vi "communication manager.vi"() -> ()   [LabVIEW 2018]
uses:
  socket SUB/socket SUB.lvclass
  C:/Users/devstaff/sparc4/s4gui/Versao ZeroMQ REQ-REP/SPARC4_GUI -v1.0.8 - com pacote communication manager/communication-manager/Socket/Socket.lvclass
  socket PUB/socket PUB.lvclass
  socket REQ/socket REQ.lvclass
  RxTx/CM_RxTx.lvclass
  <vilib>/addons/zeromq/zmq_context.lvclass
  Socket/Socket.lvclass
panel:
  in  "socket REQ":refnum<class "socket REQ.lvclass">
  out "error out":errorcluster
  in  "socket PUB.lvclass":refnum<class "socket PUB.lvclass">
  in  "socket SUB.lvclass":refnum<class "socket SUB.lvclass">
  # "Communication Manager of S4CCS"
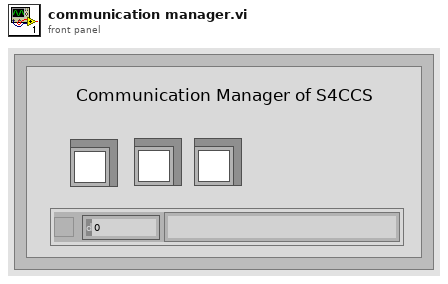
[diagram p1: front panel]
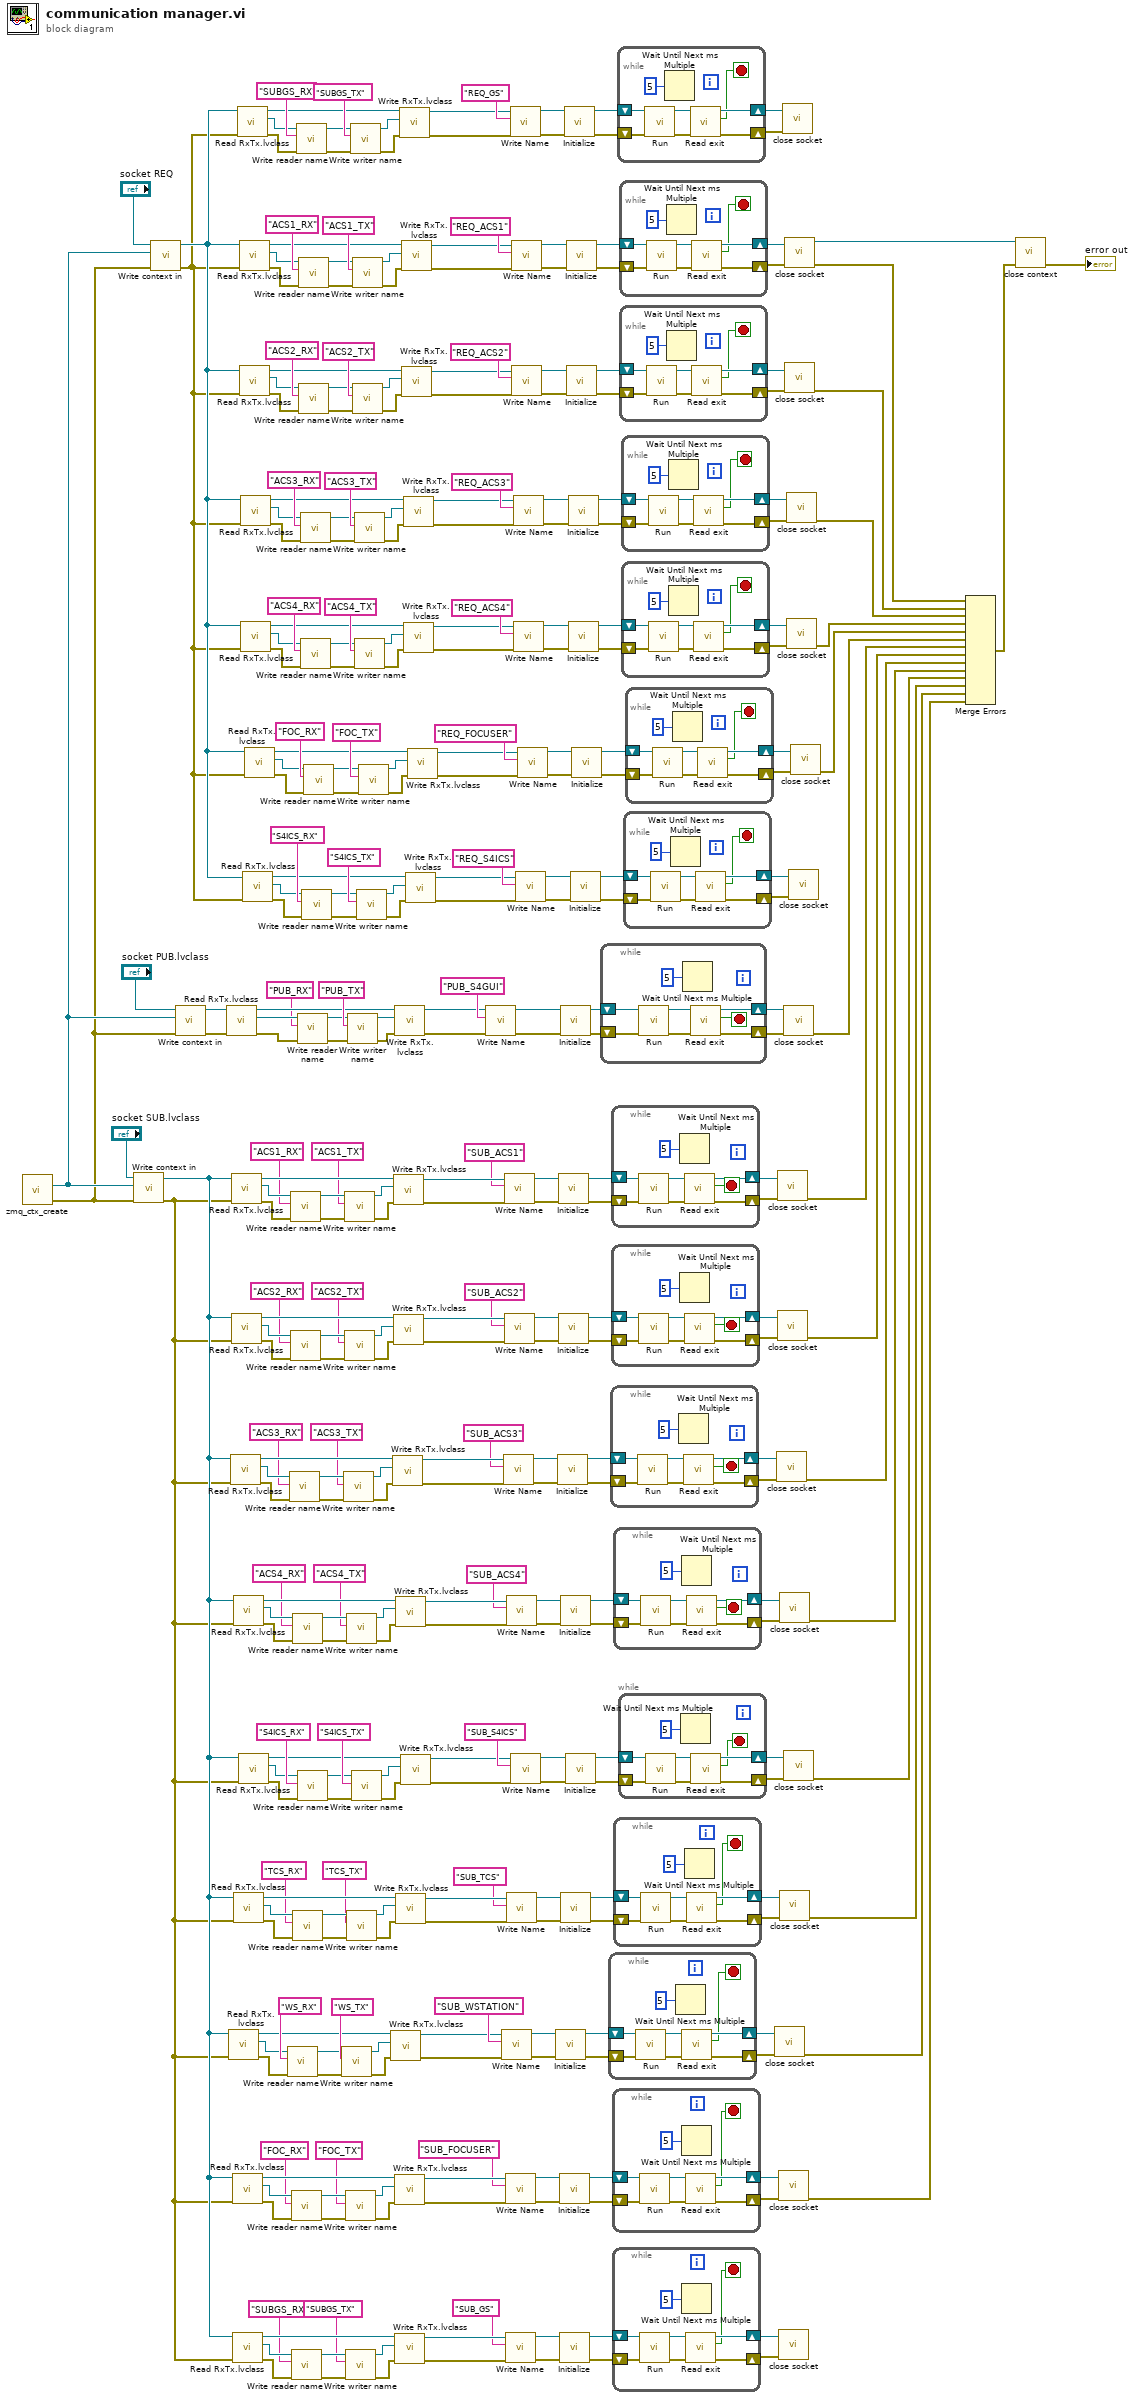
[diagram p0: block diagram]
diagram:
  n1 = call <vilib>:"zmq_ctx_create.vi"() -> ("error out"=w41:errorcluster, "context out"=w42:refnum<class "zmq_context.lvclass">)  [unwired: 4 in]
  n2 = call-dynamic "Write context in.vi"("error in (no error)"=w41, "zeromq.lvlib:ZeroMQ Context"=w42, "Socket in"="socket SUB.lvclass") -> ("error out"=w21:errorcluster, "Socket out"=w22:refnum<class "socket SUB.lvclass">)  [unwired: 7 in]
  n3 = call-dynamic "Write context in.vi"("error in (no error)"=w41, "zeromq.lvlib:ZeroMQ Context"=w42, "Socket in"="socket REQ") -> ("error out"=w1:errorcluster, "Socket out"=w2:refnum<class "socket REQ.lvclass">)  [unwired: 7 in]
  n4 = call-dynamic "Write context in.vi"("error in (no error)"=w41, "zeromq.lvlib:ZeroMQ Context"=w42, "Socket in"="socket PUB.lvclass") -> ("error out"=w199:errorcluster, "Socket out"=w200:refnum<class "socket PUB.lvclass">)  [unwired: 7 in]
  n5 = call-dynamic "Read RxTx.lvclass.vi"("error in (no error)"=w199, "Socket in"=w200) -> ("error out"=w305:errorcluster, "RxTx.lvclass"=w309:refnum<class "CM_RxTx.lvclass">, "Socket out"=w306:refnum<class "socket PUB.lvclass">)  [unwired: 7 in]
  n6 = call-dynamic "Read RxTx.lvclass.vi"("error in (no error)"=w21, "Socket in"=w22) -> ("error out"=w240:errorcluster, "RxTx.lvclass"=w244:refnum<class "CM_RxTx.lvclass">, "Socket out"=w241:refnum<class "socket SUB.lvclass">)  [unwired: 7 in]
  n7 = call-dynamic "Read RxTx.lvclass.vi"("error in (no error)"=w21, "Socket in"=w22) -> ("error out"=w109:errorcluster, "RxTx.lvclass"=w105:refnum<class "CM_RxTx.lvclass">, "Socket out"=w108:refnum<class "socket SUB.lvclass">)  [unwired: 7 in]
  n8 = call-dynamic "Read RxTx.lvclass.vi"("error in (no error)"=w21, "Socket in"=w22) -> ("error out"=w287:errorcluster, "RxTx.lvclass"=w283:refnum<class "CM_RxTx.lvclass">, "Socket out"=w286:refnum<class "socket SUB.lvclass">)  [unwired: 7 in]
  n9 = call-dynamic "Read RxTx.lvclass.vi"("error in (no error)"=w21, "Socket in"=w22) -> ("error out"=w127:errorcluster, "RxTx.lvclass"=w123:refnum<class "CM_RxTx.lvclass">, "Socket out"=w126:refnum<class "socket SUB.lvclass">)  [unwired: 7 in]
  n10 = call-dynamic "Read RxTx.lvclass.vi"("error in (no error)"=w21, "Socket in"=w22) -> ("error out"=w221:errorcluster, "RxTx.lvclass"=w217:refnum<class "CM_RxTx.lvclass">, "Socket out"=w220:refnum<class "socket SUB.lvclass">)  [unwired: 7 in]
  n11 = call-dynamic "Read RxTx.lvclass.vi"("error in (no error)"=w21, "Socket in"=w22) -> ("error out"=w31:errorcluster, "RxTx.lvclass"=w27:refnum<class "CM_RxTx.lvclass">, "Socket out"=w30:refnum<class "socket SUB.lvclass">)  [unwired: 7 in]
  n12 = call-dynamic "Read RxTx.lvclass.vi"("error in (no error)"=w21, "Socket in"=w22) -> ("error out"=w91:errorcluster, "RxTx.lvclass"=w87:refnum<class "CM_RxTx.lvclass">, "Socket out"=w90:refnum<class "socket SUB.lvclass">)  [unwired: 7 in]
  n13 = call-dynamic "Read RxTx.lvclass.vi"("error in (no error)"=w21, "Socket in"=w22) -> ("error out"=w253:errorcluster, "RxTx.lvclass"=w249:refnum<class "CM_RxTx.lvclass">, "Socket out"=w252:refnum<class "socket SUB.lvclass">)  [unwired: 7 in]
  n14 = call-dynamic "Read RxTx.lvclass.vi"("error in (no error)"=w1, "Socket in"=w2) -> ("error out"=w14:errorcluster, "RxTx.lvclass"=w18:refnum<class "CM_RxTx.lvclass">, "Socket out"=w15:refnum<class "socket REQ.lvclass">)  [unwired: 7 in]
  n15 = call-dynamic "Read RxTx.lvclass.vi"("error in (no error)"=w21, "Socket in"=w22) -> ("error out"=w272:errorcluster, "RxTx.lvclass"=w276:refnum<class "CM_RxTx.lvclass">, "Socket out"=w273:refnum<class "socket SUB.lvclass">)  [unwired: 7 in]
  n16 = call-dynamic "Read RxTx.lvclass.vi"("error in (no error)"=w1, "Socket in"=w2) -> ("error out"=w327:errorcluster, "RxTx.lvclass"=w331:refnum<class "CM_RxTx.lvclass">, "Socket out"=w328:refnum<class "socket REQ.lvclass">)  [unwired: 7 in]
  n17 = call-dynamic "Read RxTx.lvclass.vi"("error in (no error)"=w1, "Socket in"=w2) -> ("error out"=w188:errorcluster, "RxTx.lvclass"=w192:refnum<class "CM_RxTx.lvclass">, "Socket out"=w189:refnum<class "socket REQ.lvclass">)  [unwired: 7 in]
  n18 = call-dynamic "Read RxTx.lvclass.vi"("error in (no error)"=w1, "Socket in"=w2) -> ("error out"=w170:errorcluster, "RxTx.lvclass"=w174:refnum<class "CM_RxTx.lvclass">, "Socket out"=w171:refnum<class "socket REQ.lvclass">)  [unwired: 7 in]
  n19 = call-dynamic "Read RxTx.lvclass.vi"("error in (no error)"=w1, "Socket in"=w2) -> ("error out"=w152:errorcluster, "RxTx.lvclass"=w156:refnum<class "CM_RxTx.lvclass">, "Socket out"=w153:refnum<class "socket REQ.lvclass">)  [unwired: 7 in]
  n20 = call-dynamic "Read RxTx.lvclass.vi"("error in (no error)"=w1, "Socket in"=w2) -> ("error out"=w54:errorcluster, "RxTx.lvclass"=w58:refnum<class "CM_RxTx.lvclass">, "Socket out"=w55:refnum<class "socket REQ.lvclass">)  [unwired: 7 in]
  n21 = call-dynamic "Read RxTx.lvclass.vi"("error in (no error)"=w1, "Socket in"=w2) -> ("error out"=w76:errorcluster, "RxTx.lvclass"=w80:refnum<class "CM_RxTx.lvclass">, "Socket out"=w77:refnum<class "socket REQ.lvclass">)  [unwired: 7 in]
  n22 = call-dynamic "Write reader name.vi"("error in (no error)"=w240, "RX name"="WS_RX" ("reader name"), "RxTx in"=w244) -> ("error out"=w239:errorcluster, "RxTx out"=w243:refnum<class "CM_RxTx.lvclass">)  [unwired: 7 in]
  n23 = call-dynamic "Write reader name.vi"("error in (no error)"=w109, "RX name"="ACS3_RX" ("reader name"), "RxTx in"=w105) -> ("error out"=w110:errorcluster, "RxTx out"=w106:refnum<class "CM_RxTx.lvclass">)  [unwired: 7 in]
  n24 = call-dynamic "Write reader name.vi"("error in (no error)"=w287, "RX name"="ACS1_RX" ("reader name"), "RxTx in"=w283) -> ("error out"=w288:errorcluster, "RxTx out"=w284:refnum<class "CM_RxTx.lvclass">)  [unwired: 7 in]
  n25 = call-dynamic "Write reader name.vi"("error in (no error)"=w127, "RX name"="ACS2_RX" ("reader name"), "RxTx in"=w123) -> ("error out"=w128:errorcluster, "RxTx out"=w124:refnum<class "CM_RxTx.lvclass">)  [unwired: 7 in]
  n26 = call-dynamic "Write reader name.vi"("error in (no error)"=w221, "RX name"="FOC_RX" ("reader name"), "RxTx in"=w217) -> ("error out"=w222:errorcluster, "RxTx out"=w218:refnum<class "CM_RxTx.lvclass">)  [unwired: 7 in]
  n27 = call-dynamic "Write reader name.vi"("error in (no error)"=w31, "RX name"="SUBGS_RX" ("reader name"), "RxTx in"=w27) -> ("error out"=w32:errorcluster, "RxTx out"=w28:refnum<class "CM_RxTx.lvclass">)  [unwired: 7 in]
  n28 = call-dynamic "Write reader name.vi"("error in (no error)"=w91, "RX name"="ACS4_RX" ("reader name"), "RxTx in"=w87) -> ("error out"=w92:errorcluster, "RxTx out"=w88:refnum<class "CM_RxTx.lvclass">)  [unwired: 7 in]
  n29 = call-dynamic "Write reader name.vi"("error in (no error)"=w253, "RX name"="TCS_RX" ("reader name"), "RxTx in"=w249) -> ("error out"=w254:errorcluster, "RxTx out"=w250:refnum<class "CM_RxTx.lvclass">)  [unwired: 7 in]
  n30 = call-dynamic "Write reader name.vi"("error in (no error)"=w14, "RX name"="SUBGS_RX" ("reader name"), "RxTx in"=w18) -> ("error out"=w13:errorcluster, "RxTx out"=w17:refnum<class "CM_RxTx.lvclass">)  [unwired: 7 in]
  n31 = call-dynamic "Write reader name.vi"("error in (no error)"=w305, "RX name"="PUB_RX" ("reader name"), "RxTx in"=w309) -> ("error out"=w304:errorcluster, "RxTx out"=w308:refnum<class "CM_RxTx.lvclass">)  [unwired: 7 in]
  n32 = call-dynamic "Write reader name.vi"("error in (no error)"=w272, "RX name"="S4ICS_RX" ("reader name"), "RxTx in"=w276) -> ("error out"=w271:errorcluster, "RxTx out"=w275:refnum<class "CM_RxTx.lvclass">)  [unwired: 7 in]
  n33 = call-dynamic "Write reader name.vi"("error in (no error)"=w327, "RX name"="ACS1_RX" ("reader name"), "RxTx in"=w331) -> ("error out"=w326:errorcluster, "RxTx out"=w330:refnum<class "CM_RxTx.lvclass">)  [unwired: 7 in]
  n34 = call-dynamic "Write reader name.vi"("error in (no error)"=w188, "RX name"="ACS2_RX" ("reader name"), "RxTx in"=w192) -> ("error out"=w187:errorcluster, "RxTx out"=w191:refnum<class "CM_RxTx.lvclass">)  [unwired: 7 in]
  n35 = call-dynamic "Write reader name.vi"("error in (no error)"=w170, "RX name"="ACS3_RX" ("reader name"), "RxTx in"=w174) -> ("error out"=w169:errorcluster, "RxTx out"=w173:refnum<class "CM_RxTx.lvclass">)  [unwired: 7 in]
  n36 = call-dynamic "Write reader name.vi"("error in (no error)"=w152, "RX name"="ACS4_RX" ("reader name"), "RxTx in"=w156) -> ("error out"=w151:errorcluster, "RxTx out"=w155:refnum<class "CM_RxTx.lvclass">)  [unwired: 7 in]
  n37 = call-dynamic "Write reader name.vi"("error in (no error)"=w54, "RX name"="S4ICS_RX" ("reader name"), "RxTx in"=w58) -> ("error out"=w53:errorcluster, "RxTx out"=w57:refnum<class "CM_RxTx.lvclass">)  [unwired: 7 in]
  n38 = call-dynamic "Write reader name.vi"("error in (no error)"=w76, "RX name"="FOC_RX" ("reader name"), "RxTx in"=w80) -> ("error out"=w75:errorcluster, "RxTx out"=w79:refnum<class "CM_RxTx.lvclass">)  [unwired: 7 in]
  n39 = call-dynamic "Write writer name.vi"("error in (no error)"=w239, "Tx name"="WS_TX" ("writer name"), "RxTx in"=w243) -> ("error out"=w238:errorcluster, "RxTx out"=w242:refnum<class "CM_RxTx.lvclass">)  [unwired: 7 in]
  n40 = call-dynamic "Write writer name.vi"("error in (no error)"=w110, "Tx name"="ACS3_TX" ("writer name"), "RxTx in"=w106) -> ("error out"=w111:errorcluster, "RxTx out"=w107:refnum<class "CM_RxTx.lvclass">)  [unwired: 7 in]
  n41 = call-dynamic "Write writer name.vi"("error in (no error)"=w288, "Tx name"="ACS1_TX" ("writer name"), "RxTx in"=w284) -> ("error out"=w289:errorcluster, "RxTx out"=w285:refnum<class "CM_RxTx.lvclass">)  [unwired: 7 in]
  n42 = call-dynamic "Write writer name.vi"("error in (no error)"=w128, "Tx name"="ACS2_TX" ("writer name"), "RxTx in"=w124) -> ("error out"=w129:errorcluster, "RxTx out"=w125:refnum<class "CM_RxTx.lvclass">)  [unwired: 7 in]
  n43 = call-dynamic "Write writer name.vi"("error in (no error)"=w222, "Tx name"="FOC_TX" ("writer name"), "RxTx in"=w218) -> ("error out"=w223:errorcluster, "RxTx out"=w219:refnum<class "CM_RxTx.lvclass">)  [unwired: 7 in]
  n44 = call-dynamic "Write writer name.vi"("error in (no error)"=w32, "Tx name"="SUBGS_TX" ("writer name"), "RxTx in"=w28) -> ("error out"=w33:errorcluster, "RxTx out"=w29:refnum<class "CM_RxTx.lvclass">)  [unwired: 7 in]
  n45 = call-dynamic "Write writer name.vi"("error in (no error)"=w92, "Tx name"="ACS4_TX" ("writer name"), "RxTx in"=w88) -> ("error out"=w93:errorcluster, "RxTx out"=w89:refnum<class "CM_RxTx.lvclass">)  [unwired: 7 in]
  n46 = call-dynamic "Write writer name.vi"("error in (no error)"=w254, "Tx name"="TCS_TX" ("writer name"), "RxTx in"=w250) -> ("error out"=w255:errorcluster, "RxTx out"=w251:refnum<class "CM_RxTx.lvclass">)  [unwired: 7 in]
  n47 = call-dynamic "Write writer name.vi"("error in (no error)"=w304, "Tx name"="PUB_TX" ("writer name"), "RxTx in"=w308) -> ("error out"=w303:errorcluster, "RxTx out"=w307:refnum<class "CM_RxTx.lvclass">)  [unwired: 7 in]
  n48 = call-dynamic "Write writer name.vi"("error in (no error)"=w13, "Tx name"="SUBGS_TX" ("writer name"), "RxTx in"=w17) -> ("error out"=w12:errorcluster, "RxTx out"=w16:refnum<class "CM_RxTx.lvclass">)  [unwired: 7 in]
  n49 = call-dynamic "Write writer name.vi"("error in (no error)"=w271, "Tx name"="S4ICS_TX" ("writer name"), "RxTx in"=w275) -> ("error out"=w270:errorcluster, "RxTx out"=w274:refnum<class "CM_RxTx.lvclass">)  [unwired: 7 in]
  n50 = call-dynamic "Write writer name.vi"("error in (no error)"=w326, "Tx name"="ACS1_TX" ("writer name"), "RxTx in"=w330) -> ("error out"=w325:errorcluster, "RxTx out"=w329:refnum<class "CM_RxTx.lvclass">)  [unwired: 7 in]
  n51 = call-dynamic "Write writer name.vi"("error in (no error)"=w187, "Tx name"="ACS2_TX" ("writer name"), "RxTx in"=w191) -> ("error out"=w186:errorcluster, "RxTx out"=w190:refnum<class "CM_RxTx.lvclass">)  [unwired: 7 in]
  n52 = call-dynamic "Write writer name.vi"("error in (no error)"=w169, "Tx name"="ACS3_TX" ("writer name"), "RxTx in"=w173) -> ("error out"=w168:errorcluster, "RxTx out"=w172:refnum<class "CM_RxTx.lvclass">)  [unwired: 7 in]
  n53 = call-dynamic "Write writer name.vi"("error in (no error)"=w151, "Tx name"="ACS4_TX" ("writer name"), "RxTx in"=w155) -> ("error out"=w150:errorcluster, "RxTx out"=w154:refnum<class "CM_RxTx.lvclass">)  [unwired: 7 in]
  n54 = call-dynamic "Write writer name.vi"("error in (no error)"=w53, "Tx name"="S4ICS_TX" ("writer name"), "RxTx in"=w57) -> ("error out"=w52:errorcluster, "RxTx out"=w56:refnum<class "CM_RxTx.lvclass">)  [unwired: 7 in]
  n55 = call-dynamic "Write writer name.vi"("error in (no error)"=w75, "Tx name"="FOC_TX" ("writer name"), "RxTx in"=w79) -> ("error out"=w74:errorcluster, "RxTx out"=w78:refnum<class "CM_RxTx.lvclass">)  [unwired: 7 in]
  n56 = call-dynamic "Write RxTx.lvclass.vi"("error in (no error)"=w238, "RxTx.lvclass"=w242, "Socket in"=w241) -> ("error out"=w235:errorcluster, "Socket out"=w236:refnum<class "socket SUB.lvclass">)  [unwired: 7 in]
  n57 = call-dynamic "Write RxTx.lvclass.vi"("error in (no error)"=w111, "RxTx.lvclass"=w107, "Socket in"=w108) -> ("error out"=w114:errorcluster, "Socket out"=w113:refnum<class "socket SUB.lvclass">)  [unwired: 7 in]
  n58 = call-dynamic "Write RxTx.lvclass.vi"("error in (no error)"=w289, "RxTx.lvclass"=w285, "Socket in"=w286) -> ("error out"=w292:errorcluster, "Socket out"=w291:refnum<class "socket SUB.lvclass">)  [unwired: 7 in]
  n59 = call-dynamic "Write RxTx.lvclass.vi"("error in (no error)"=w129, "RxTx.lvclass"=w125, "Socket in"=w126) -> ("error out"=w132:errorcluster, "Socket out"=w131:refnum<class "socket SUB.lvclass">)  [unwired: 7 in]
  n60 = call-dynamic "Write RxTx.lvclass.vi"("error in (no error)"=w303, "RxTx.lvclass"=w307, "Socket in"=w306) -> ("error out"=w201:errorcluster, "Socket out"=w202:refnum<class "socket PUB.lvclass">)  [unwired: 7 in]
  n61 = call-dynamic "Write RxTx.lvclass.vi"("error in (no error)"=w223, "RxTx.lvclass"=w219, "Socket in"=w220) -> ("error out"=w226:errorcluster, "Socket out"=w225:refnum<class "socket SUB.lvclass">)  [unwired: 7 in]
  n62 = call-dynamic "Write RxTx.lvclass.vi"("error in (no error)"=w33, "RxTx.lvclass"=w29, "Socket in"=w30) -> ("error out"=w36:errorcluster, "Socket out"=w35:refnum<class "socket SUB.lvclass">)  [unwired: 7 in]
  n63 = call-dynamic "Write RxTx.lvclass.vi"("error in (no error)"=w93, "RxTx.lvclass"=w89, "Socket in"=w90) -> ("error out"=w96:errorcluster, "Socket out"=w95:refnum<class "socket SUB.lvclass">)  [unwired: 7 in]
  n64 = call-dynamic "Write RxTx.lvclass.vi"("error in (no error)"=w255, "RxTx.lvclass"=w251, "Socket in"=w252) -> ("error out"=w258:errorcluster, "Socket out"=w257:refnum<class "socket SUB.lvclass">)  [unwired: 7 in]
  n65 = call-dynamic "Write RxTx.lvclass.vi"("error in (no error)"=w12, "RxTx.lvclass"=w16, "Socket in"=w15) -> ("error out"=w9:errorcluster, "Socket out"=w10:refnum<class "socket REQ.lvclass">)  [unwired: 7 in]
  n66 = call-dynamic "Write RxTx.lvclass.vi"("error in (no error)"=w270, "RxTx.lvclass"=w274, "Socket in"=w273) -> ("error out"=w267:errorcluster, "Socket out"=w268:refnum<class "socket SUB.lvclass">)  [unwired: 7 in]
  n67 = call-dynamic "Write RxTx.lvclass.vi"("error in (no error)"=w325, "RxTx.lvclass"=w329, "Socket in"=w328) -> ("error out"=w322:errorcluster, "Socket out"=w323:refnum<class "socket REQ.lvclass">)  [unwired: 7 in]
  n68 = call-dynamic "Write RxTx.lvclass.vi"("error in (no error)"=w186, "RxTx.lvclass"=w190, "Socket in"=w189) -> ("error out"=w183:errorcluster, "Socket out"=w184:refnum<class "socket REQ.lvclass">)  [unwired: 7 in]
  n69 = call-dynamic "Write RxTx.lvclass.vi"("error in (no error)"=w168, "RxTx.lvclass"=w172, "Socket in"=w171) -> ("error out"=w165:errorcluster, "Socket out"=w166:refnum<class "socket REQ.lvclass">)  [unwired: 7 in]
  n70 = call-dynamic "Write RxTx.lvclass.vi"("error in (no error)"=w150, "RxTx.lvclass"=w154, "Socket in"=w153) -> ("error out"=w147:errorcluster, "Socket out"=w148:refnum<class "socket REQ.lvclass">)  [unwired: 7 in]
  n71 = call-dynamic "Write RxTx.lvclass.vi"("error in (no error)"=w52, "RxTx.lvclass"=w56, "Socket in"=w55) -> ("error out"=w49:errorcluster, "Socket out"=w50:refnum<class "socket REQ.lvclass">)  [unwired: 7 in]
  n72 = call-dynamic "Write RxTx.lvclass.vi"("error in (no error)"=w74, "RxTx.lvclass"=w78, "Socket in"=w77) -> ("error out"=w71:errorcluster, "Socket out"=w72:refnum<class "socket REQ.lvclass">)  [unwired: 7 in]
  n73 = call-dynamic "Write Name.vi"("error in (no error)"=w201, "Name"="PUB_S4GUI", "Socket in"=w202) -> ("error out"=w301:errorcluster, "Socket out"=w302:refnum<class "socket PUB.lvclass">)  [unwired: 7 in]
  n74 = call-dynamic "Write Name.vi"("error in (no error)"=w235, "Name"="SUB_WSTATION", "Socket in"=w236) -> ("error out"=w209:errorcluster, "Socket out"=w210:refnum<class "socket SUB.lvclass">)  [unwired: 7 in]
  n75 = call-dynamic "Write Name.vi"("error in (no error)"=w114, "Name"="SUB_ACS3", "Socket in"=w113) -> ("error out"=w101:errorcluster, "Socket out"=w102:refnum<class "socket SUB.lvclass">)  [unwired: 7 in]
  n76 = call-dynamic "Write Name.vi"("error in (no error)"=w292, "Name"="SUB_ACS1", "Socket in"=w291) -> ("error out"=w207:errorcluster, "Socket out"=w208:refnum<class "socket SUB.lvclass">)  [unwired: 7 in]
  n77 = call-dynamic "Write Name.vi"("error in (no error)"=w132, "Name"="SUB_ACS2", "Socket in"=w131) -> ("error out"=w119:errorcluster, "Socket out"=w120:refnum<class "socket SUB.lvclass">)  [unwired: 7 in]
  n78 = call-dynamic "Write Name.vi"("error in (no error)"=w226, "Name"="SUB_FOCUSER", "Socket in"=w225) -> ("error out"=w203:errorcluster, "Socket out"=w204:refnum<class "socket SUB.lvclass">)  [unwired: 7 in]
  n79 = call-dynamic "Write Name.vi"("error in (no error)"=w36, "Name"="SUB_GS", "Socket in"=w35) -> ("error out"=w23:errorcluster, "Socket out"=w24:refnum<class "socket SUB.lvclass">)  [unwired: 7 in]
  n80 = call-dynamic "Write Name.vi"("error in (no error)"=w96, "Name"="SUB_ACS4", "Socket in"=w95) -> ("error out"=w83:errorcluster, "Socket out"=w84:refnum<class "socket SUB.lvclass">)  [unwired: 7 in]
  n81 = call-dynamic "Write Name.vi"("error in (no error)"=w258, "Name"="SUB_TCS", "Socket in"=w257) -> ("error out"=w213:errorcluster, "Socket out"=w214:refnum<class "socket SUB.lvclass">)  [unwired: 7 in]
  n82 = call-dynamic "Write Name.vi"("error in (no error)"=w9, "Name"="REQ_GS", "Socket in"=w10) -> ("error out"=w4:errorcluster, "Socket out"=w5:refnum<class "socket REQ.lvclass">)  [unwired: 7 in]
  n83 = call-dynamic "Write Name.vi"("error in (no error)"=w267, "Name"="SUB_S4ICS", "Socket in"=w268) -> ("error out"=w211:errorcluster, "Socket out"=w212:refnum<class "socket SUB.lvclass">)  [unwired: 7 in]
  n84 = call-dynamic "Write Name.vi"("error in (no error)"=w322, "Name"="REQ_ACS1", "Socket in"=w323) -> ("error out"=w205:errorcluster, "Socket out"=w206:refnum<class "socket REQ.lvclass">)  [unwired: 7 in]
  n85 = call-dynamic "Write Name.vi"("error in (no error)"=w183, "Name"="REQ_ACS2", "Socket in"=w184) -> ("error out"=w178:errorcluster, "Socket out"=w179:refnum<class "socket REQ.lvclass">)  [unwired: 7 in]
  n86 = call-dynamic "Write Name.vi"("error in (no error)"=w165, "Name"="REQ_ACS3", "Socket in"=w166) -> ("error out"=w160:errorcluster, "Socket out"=w161:refnum<class "socket REQ.lvclass">)  [unwired: 7 in]
  n87 = call-dynamic "Write Name.vi"("error in (no error)"=w147, "Name"="REQ_ACS4", "Socket in"=w148) -> ("error out"=w142:errorcluster, "Socket out"=w143:refnum<class "socket REQ.lvclass">)  [unwired: 7 in]
  n88 = call-dynamic "Write Name.vi"("error in (no error)"=w49, "Name"="REQ_S4ICS", "Socket in"=w50) -> ("error out"=w44:errorcluster, "Socket out"=w45:refnum<class "socket REQ.lvclass">)  [unwired: 7 in]
  n89 = call-dynamic "Write Name.vi"("error in (no error)"=w71, "Name"="REQ_FOCUSER", "Socket in"=w72) -> ("error out"=w66:errorcluster, "Socket out"=w67:refnum<class "socket REQ.lvclass">)  [unwired: 7 in]
  n90 = call-dynamic "Initialize.vi"("error in (no error)"=w209, "socket SUB in"=w210) -> ("error out"=w232:errorcluster, "socket SUB out"=w234:refnum<class "socket SUB.lvclass">)  [unwired: 8 in]
  n91 = call-dynamic "Initialize.vi"("error in (no error)"=w101, "socket SUB in"=w102) -> ("error out"=w117:errorcluster, "socket SUB out"=w115:refnum<class "socket SUB.lvclass">)  [unwired: 8 in]
  n92 = call-dynamic "Initialize.vi"("error in (no error)"=w207, "socket SUB in"=w208) -> ("error out"=w295:errorcluster, "socket SUB out"=w293:refnum<class "socket SUB.lvclass">)  [unwired: 8 in]
  n93 = call-dynamic "Initialize.vi"("error in (no error)"=w119, "socket SUB in"=w120) -> ("error out"=w135:errorcluster, "socket SUB out"=w133:refnum<class "socket SUB.lvclass">)  [unwired: 8 in]
  n94 = call-dynamic "Initialize.vi"("error in (no error)"=w203, "socket SUB in"=w204) -> ("error out"=w229:errorcluster, "socket SUB out"=w227:refnum<class "socket SUB.lvclass">)  [unwired: 8 in]
  n95 = call-dynamic "Initialize.vi"("error in (no error)"=w23, "socket SUB in"=w24) -> ("error out"=w39:errorcluster, "socket SUB out"=w37:refnum<class "socket SUB.lvclass">)  [unwired: 8 in]
  n96 = call-dynamic "Initialize.vi"("error in (no error)"=w301, "socket PUB in"=w302) -> ("error out"=w298:errorcluster, "socket PUB out"=w300:refnum<class "socket PUB.lvclass">)  [unwired: 8 in]
  n97 = call-dynamic "Initialize.vi"("error in (no error)"=w83, "socket SUB in"=w84) -> ("error out"=w99:errorcluster, "socket SUB out"=w97:refnum<class "socket SUB.lvclass">)  [unwired: 8 in]
  n98 = call-dynamic "Initialize.vi"("error in (no error)"=w213, "socket SUB in"=w214) -> ("error out"=w261:errorcluster, "socket SUB out"=w259:refnum<class "socket SUB.lvclass">)  [unwired: 8 in]
  n99 = call-dynamic "Initialize.vi"("error in (no error)"=w4, "socket REQ in"=w5) -> ("error out"=w3:errorcluster, "socket REQ out"=w8:refnum<class "socket REQ.lvclass">)  [unwired: 8 in]
  n100 = call-dynamic "Initialize.vi"("error in (no error)"=w211, "socket SUB in"=w212) -> ("error out"=w264:errorcluster, "socket SUB out"=w266:refnum<class "socket SUB.lvclass">)  [unwired: 8 in]
  n101 = call-dynamic "Initialize.vi"("error in (no error)"=w205, "socket REQ in"=w206) -> ("error out"=w196:errorcluster, "socket REQ out"=w321:refnum<class "socket REQ.lvclass">)  [unwired: 8 in]
  n102 = call-dynamic "Initialize.vi"("error in (no error)"=w178, "socket REQ in"=w179) -> ("error out"=w177:errorcluster, "socket REQ out"=w182:refnum<class "socket REQ.lvclass">)  [unwired: 8 in]
  n103 = call-dynamic "Initialize.vi"("error in (no error)"=w160, "socket REQ in"=w161) -> ("error out"=w159:errorcluster, "socket REQ out"=w164:refnum<class "socket REQ.lvclass">)  [unwired: 8 in]
  n104 = call-dynamic "Initialize.vi"("error in (no error)"=w142, "socket REQ in"=w143) -> ("error out"=w141:errorcluster, "socket REQ out"=w146:refnum<class "socket REQ.lvclass">)  [unwired: 8 in]
  n105 = call-dynamic "Initialize.vi"("error in (no error)"=w44, "socket REQ in"=w45) -> ("error out"=w43:errorcluster, "socket REQ out"=w48:refnum<class "socket REQ.lvclass">)  [unwired: 8 in]
  n106 = call-dynamic "Initialize.vi"("error in (no error)"=w66, "socket REQ in"=w67) -> ("error out"=w65:errorcluster, "socket REQ out"=w70:refnum<class "socket REQ.lvclass">)  [unwired: 8 in]
  n107 = while {
    shift-right: [w338] -> w299
    shift-left: w300 -> [w342]
    shift-right: [w337] -> w297
    shift-left: w298 -> [w341]
    stop <- w336 stop-if-true
    n108 = call-dynamic "Run.vi"("error in (no error)"=w341, "socket PUB in"=w342) -> ("error out"=w340:errorcluster, "socket PUB out"=w339:refnum<class "socket PUB.lvclass">)  [unwired: 8 in]
    n109 = Wait Until Next ms Multiple(millisecond multiple=u32 5) -> ()  [unwired: 1 out]
    n110 = call-dynamic "Read exit.vi"("error in (no error)"=w340, "Socket in"=w339) -> ("error out"=w337:errorcluster, "exit"=w336:bool, "Socket out"=w338:refnum<class "socket PUB.lvclass">)  [unwired: 7 in]
  }
  n111 = while {
    shift-right: [w348] -> w233
    shift-left: w234 -> [w350]
    shift-right: [w345] -> w231
    shift-left: w232 -> [w347]
    stop <- w344 stop-if-true
    n112 = call-dynamic "Run.vi"("error in (no error)"=w347, "socket SUB in"=w350) -> ("error out"=w346:errorcluster, "socket SUB out"=w349:refnum<class "socket SUB.lvclass">)  [unwired: 8 in]
    n113 = Wait Until Next ms Multiple(millisecond multiple=u32 5) -> ()  [unwired: 1 out]
    n114 = call-dynamic "Read exit.vi"("error in (no error)"=w346, "Socket in"=w349) -> ("error out"=w345:errorcluster, "exit"=w344:bool, "Socket out"=w348:refnum<class "socket SUB.lvclass">)  [unwired: 7 in]
  }
  n115 = while {
    shift-right: [w356] -> w116
    shift-left: w115 -> [w358]
    shift-right: [w353] -> w118
    shift-left: w117 -> [w355]
    stop <- w352 stop-if-true
    n116 = call-dynamic "Run.vi"("error in (no error)"=w355, "socket SUB in"=w358) -> ("error out"=w354:errorcluster, "socket SUB out"=w357:refnum<class "socket SUB.lvclass">)  [unwired: 8 in]
    n117 = Wait Until Next ms Multiple(millisecond multiple=u32 5) -> ()  [unwired: 1 out]
    n118 = call-dynamic "Read exit.vi"("error in (no error)"=w354, "Socket in"=w357) -> ("error out"=w353:errorcluster, "exit"=w352:bool, "Socket out"=w356:refnum<class "socket SUB.lvclass">)  [unwired: 7 in]
  }
  n119 = while {
    shift-right: [w364] -> w294
    shift-left: w293 -> [w366]
    shift-right: [w361] -> w296
    shift-left: w295 -> [w363]
    stop <- w360 stop-if-true
    n120 = call-dynamic "Run.vi"("error in (no error)"=w363, "socket SUB in"=w366) -> ("error out"=w362:errorcluster, "socket SUB out"=w365:refnum<class "socket SUB.lvclass">)  [unwired: 8 in]
    n121 = Wait Until Next ms Multiple(millisecond multiple=u32 5) -> ()  [unwired: 1 out]
    n122 = call-dynamic "Read exit.vi"("error in (no error)"=w362, "Socket in"=w365) -> ("error out"=w361:errorcluster, "exit"=w360:bool, "Socket out"=w364:refnum<class "socket SUB.lvclass">)  [unwired: 7 in]
  }
  n123 = while {
    shift-right: [w372] -> w134
    shift-left: w133 -> [w374]
    shift-right: [w369] -> w136
    shift-left: w135 -> [w371]
    stop <- w368 stop-if-true
    n124 = call-dynamic "Run.vi"("error in (no error)"=w371, "socket SUB in"=w374) -> ("error out"=w370:errorcluster, "socket SUB out"=w373:refnum<class "socket SUB.lvclass">)  [unwired: 8 in]
    n125 = Wait Until Next ms Multiple(millisecond multiple=u32 5) -> ()  [unwired: 1 out]
    n126 = call-dynamic "Read exit.vi"("error in (no error)"=w370, "Socket in"=w373) -> ("error out"=w369:errorcluster, "exit"=w368:bool, "Socket out"=w372:refnum<class "socket SUB.lvclass">)  [unwired: 7 in]
  }
  n127 = while {
    shift-right: [w380] -> w228
    shift-left: w227 -> [w382]
    shift-right: [w377] -> w230
    shift-left: w229 -> [w379]
    stop <- w376 stop-if-true
    n128 = call-dynamic "Run.vi"("error in (no error)"=w379, "socket SUB in"=w382) -> ("error out"=w378:errorcluster, "socket SUB out"=w381:refnum<class "socket SUB.lvclass">)  [unwired: 8 in]
    n129 = Wait Until Next ms Multiple(millisecond multiple=u32 5) -> ()  [unwired: 1 out]
    n130 = call-dynamic "Read exit.vi"("error in (no error)"=w378, "Socket in"=w381) -> ("error out"=w377:errorcluster, "exit"=w376:bool, "Socket out"=w380:refnum<class "socket SUB.lvclass">)  [unwired: 7 in]
  }
  n131 = while {
    shift-right: [w388] -> w38
    shift-left: w37 -> [w390]
    shift-right: [w385] -> w40
    shift-left: w39 -> [w387]
    stop <- w384 stop-if-true
    n132 = call-dynamic "Run.vi"("error in (no error)"=w387, "socket SUB in"=w390) -> ("error out"=w386:errorcluster, "socket SUB out"=w389:refnum<class "socket SUB.lvclass">)  [unwired: 8 in]
    n133 = Wait Until Next ms Multiple(millisecond multiple=u32 5) -> ()  [unwired: 1 out]
    n134 = call-dynamic "Read exit.vi"("error in (no error)"=w386, "Socket in"=w389) -> ("error out"=w385:errorcluster, "exit"=w384:bool, "Socket out"=w388:refnum<class "socket SUB.lvclass">)  [unwired: 7 in]
  }
  n135 = while {
    shift-right: [w396] -> w98
    shift-left: w97 -> [w398]
    shift-right: [w393] -> w100
    shift-left: w99 -> [w395]
    stop <- w392 stop-if-true
    n136 = call-dynamic "Run.vi"("error in (no error)"=w395, "socket SUB in"=w398) -> ("error out"=w394:errorcluster, "socket SUB out"=w397:refnum<class "socket SUB.lvclass">)  [unwired: 8 in]
    n137 = Wait Until Next ms Multiple(millisecond multiple=u32 5) -> ()  [unwired: 1 out]
    n138 = call-dynamic "Read exit.vi"("error in (no error)"=w394, "Socket in"=w397) -> ("error out"=w393:errorcluster, "exit"=w392:bool, "Socket out"=w396:refnum<class "socket SUB.lvclass">)  [unwired: 7 in]
  }
  n139 = while {
    shift-right: [w404] -> w260
    shift-left: w259 -> [w406]
    shift-right: [w401] -> w262
    shift-left: w261 -> [w403]
    stop <- w400 stop-if-true
    n140 = call-dynamic "Run.vi"("error in (no error)"=w403, "socket SUB in"=w406) -> ("error out"=w402:errorcluster, "socket SUB out"=w405:refnum<class "socket SUB.lvclass">)  [unwired: 8 in]
    n141 = Wait Until Next ms Multiple(millisecond multiple=u32 5) -> ()  [unwired: 1 out]
    n142 = call-dynamic "Read exit.vi"("error in (no error)"=w402, "Socket in"=w405) -> ("error out"=w401:errorcluster, "exit"=w400:bool, "Socket out"=w404:refnum<class "socket SUB.lvclass">)  [unwired: 7 in]
  }
  n143 = while {
    shift-right: [w412] -> w7
    shift-left: w8 -> [w414]
    shift-right: [w409] -> w6
    shift-left: w3 -> [w411]
    stop <- w408 stop-if-true
    n144 = call-dynamic "Run.vi"("error in (no error)"=w411, "socket REQ in"=w414) -> ("error out"=w410:errorcluster, "socket REQ out"=w413:refnum<class "socket REQ.lvclass">)  [unwired: 8 in]
    n145 = Wait Until Next ms Multiple(millisecond multiple=u32 5) -> ()  [unwired: 1 out]
    n146 = call-dynamic "Read exit.vi"("error in (no error)"=w410, "Socket in"=w413) -> ("error out"=w409:errorcluster, "exit"=w408:bool, "Socket out"=w412:refnum<class "socket REQ.lvclass">)  [unwired: 7 in]
  }
  n147 = while {
    shift-right: [w420] -> w265
    shift-left: w266 -> [w422]
    shift-right: [w417] -> w263
    shift-left: w264 -> [w419]
    stop <- w416 stop-if-true
    n148 = call-dynamic "Run.vi"("error in (no error)"=w419, "socket SUB in"=w422) -> ("error out"=w418:errorcluster, "socket SUB out"=w421:refnum<class "socket SUB.lvclass">)  [unwired: 8 in]
    n149 = Wait Until Next ms Multiple(millisecond multiple=u32 5) -> ()  [unwired: 1 out]
    n150 = call-dynamic "Read exit.vi"("error in (no error)"=w418, "Socket in"=w421) -> ("error out"=w417:errorcluster, "exit"=w416:bool, "Socket out"=w420:refnum<class "socket SUB.lvclass">)  [unwired: 7 in]
  }
  n151 = while {
    shift-right: [w428] -> w320
    shift-left: w321 -> [w430]
    shift-right: [w425] -> w319
    shift-left: w196 -> [w427]
    stop <- w424 stop-if-true
    n152 = call-dynamic "Run.vi"("error in (no error)"=w427, "socket REQ in"=w430) -> ("error out"=w426:errorcluster, "socket REQ out"=w429:refnum<class "socket REQ.lvclass">)  [unwired: 8 in]
    n153 = Wait Until Next ms Multiple(millisecond multiple=u32 5) -> ()  [unwired: 1 out]
    n154 = call-dynamic "Read exit.vi"("error in (no error)"=w426, "Socket in"=w429) -> ("error out"=w425:errorcluster, "exit"=w424:bool, "Socket out"=w428:refnum<class "socket REQ.lvclass">)  [unwired: 7 in]
  }
  n155 = while {
    shift-right: [w436] -> w181
    shift-left: w182 -> [w438]
    shift-right: [w433] -> w180
    shift-left: w177 -> [w435]
    stop <- w432 stop-if-true
    n156 = call-dynamic "Run.vi"("error in (no error)"=w435, "socket REQ in"=w438) -> ("error out"=w434:errorcluster, "socket REQ out"=w437:refnum<class "socket REQ.lvclass">)  [unwired: 8 in]
    n157 = Wait Until Next ms Multiple(millisecond multiple=u32 5) -> ()  [unwired: 1 out]
    n158 = call-dynamic "Read exit.vi"("error in (no error)"=w434, "Socket in"=w437) -> ("error out"=w433:errorcluster, "exit"=w432:bool, "Socket out"=w436:refnum<class "socket REQ.lvclass">)  [unwired: 7 in]
  }
  n159 = while {
    shift-right: [w444] -> w163
    shift-left: w164 -> [w446]
    shift-right: [w441] -> w162
    shift-left: w159 -> [w443]
    stop <- w440 stop-if-true
    n160 = call-dynamic "Run.vi"("error in (no error)"=w443, "socket REQ in"=w446) -> ("error out"=w442:errorcluster, "socket REQ out"=w445:refnum<class "socket REQ.lvclass">)  [unwired: 8 in]
    n161 = Wait Until Next ms Multiple(millisecond multiple=u32 5) -> ()  [unwired: 1 out]
    n162 = call-dynamic "Read exit.vi"("error in (no error)"=w442, "Socket in"=w445) -> ("error out"=w441:errorcluster, "exit"=w440:bool, "Socket out"=w444:refnum<class "socket REQ.lvclass">)  [unwired: 7 in]
  }
  n163 = while {
    shift-right: [w452] -> w145
    shift-left: w146 -> [w454]
    shift-right: [w449] -> w144
    shift-left: w141 -> [w451]
    stop <- w448 stop-if-true
    n164 = call-dynamic "Run.vi"("error in (no error)"=w451, "socket REQ in"=w454) -> ("error out"=w450:errorcluster, "socket REQ out"=w453:refnum<class "socket REQ.lvclass">)  [unwired: 8 in]
    n165 = Wait Until Next ms Multiple(millisecond multiple=u32 5) -> ()  [unwired: 1 out]
    n166 = call-dynamic "Read exit.vi"("error in (no error)"=w450, "Socket in"=w453) -> ("error out"=w449:errorcluster, "exit"=w448:bool, "Socket out"=w452:refnum<class "socket REQ.lvclass">)  [unwired: 7 in]
  }
  n167 = while {
    shift-right: [w460] -> w47
    shift-left: w48 -> [w462]
    shift-right: [w457] -> w46
    shift-left: w43 -> [w459]
    stop <- w456 stop-if-true
    n168 = call-dynamic "Run.vi"("error in (no error)"=w459, "socket REQ in"=w462) -> ("error out"=w458:errorcluster, "socket REQ out"=w461:refnum<class "socket REQ.lvclass">)  [unwired: 8 in]
    n169 = Wait Until Next ms Multiple(millisecond multiple=u32 5) -> ()  [unwired: 1 out]
    n170 = call-dynamic "Read exit.vi"("error in (no error)"=w458, "Socket in"=w461) -> ("error out"=w457:errorcluster, "exit"=w456:bool, "Socket out"=w460:refnum<class "socket REQ.lvclass">)  [unwired: 7 in]
  }
  n171 = while {
    shift-right: [w468] -> w69
    shift-left: w70 -> [w470]
    shift-right: [w465] -> w68
    shift-left: w65 -> [w467]
    stop <- w464 stop-if-true
    n172 = call-dynamic "Run.vi"("error in (no error)"=w467, "socket REQ in"=w470) -> ("error out"=w466:errorcluster, "socket REQ out"=w469:refnum<class "socket REQ.lvclass">)  [unwired: 8 in]
    n173 = Wait Until Next ms Multiple(millisecond multiple=u32 5) -> ()  [unwired: 1 out]
    n174 = call-dynamic "Read exit.vi"("error in (no error)"=w466, "Socket in"=w469) -> ("error out"=w465:errorcluster, "exit"=w464:bool, "Socket out"=w468:refnum<class "socket REQ.lvclass">)  [unwired: 7 in]
  }
  n175 = call "close socket.vi"("error in (no error)"=w231, "Socket in"=w233) -> ("error out"=w311:errorcluster)  [unwired: 8 in, 1 out]
  n176 = call "close socket.vi"("error in (no error)"=w118, "Socket in"=w116) -> ("error out"=w62:errorcluster)  [unwired: 8 in, 1 out]
  n177 = call "close socket.vi"("error in (no error)"=w296, "Socket in"=w294) -> ("error out"=w317:errorcluster)  [unwired: 8 in, 1 out]
  n178 = call "close socket.vi"("error in (no error)"=w136, "Socket in"=w134) -> ("error out"=w63:errorcluster)  [unwired: 8 in, 1 out]
  n179 = call "close socket.vi"("error in (no error)"=w230, "Socket in"=w228) -> ("error out"=w310:errorcluster)  [unwired: 8 in, 1 out]
  n180 = call "close socket.vi"("error in (no error)"=w40, "Socket in"=w38) -> ()  [unwired: 8 in, 2 out]
  n181 = call "close socket.vi"("error in (no error)"=w100, "Socket in"=w98) -> ("error out"=w61:errorcluster)  [unwired: 8 in, 1 out]
  n182 = call "close socket.vi"("error in (no error)"=w262, "Socket in"=w260) -> ("error out"=w312:errorcluster)  [unwired: 8 in, 1 out]
  n183 = call "close socket.vi"("error in (no error)"=w6, "Socket in"=w7) -> ()  [unwired: 8 in, 2 out]
  n184 = call "close socket.vi"("error in (no error)"=w297, "Socket in"=w299) -> ("error out"=w318:errorcluster)  [unwired: 8 in, 1 out]
  n185 = call "close socket.vi"("error in (no error)"=w263, "Socket in"=w265) -> ("error out"=w313:errorcluster)  [unwired: 8 in, 1 out]
  n186 = call "close socket.vi"("error in (no error)"=w319, "Socket in"=w320) -> ("error out"=w140:errorcluster, "Socket out"=w315:refnum<class "socket REQ.lvclass">)  [unwired: 8 in]
  n187 = call "close socket.vi"("error in (no error)"=w180, "Socket in"=w181) -> ("error out"=w139:errorcluster)  [unwired: 8 in, 1 out]
  n188 = call "close socket.vi"("error in (no error)"=w162, "Socket in"=w163) -> ("error out"=w138:errorcluster)  [unwired: 8 in, 1 out]
  n189 = call "close socket.vi"("error in (no error)"=w144, "Socket in"=w145) -> ("error out"=w137:errorcluster)  [unwired: 8 in, 1 out]
  n190 = call "close socket.vi"("error in (no error)"=w46, "Socket in"=w47) -> ()  [unwired: 8 in, 2 out]
  n191 = call "close socket.vi"("error in (no error)"=w68, "Socket in"=w69) -> ("error out"=w64:errorcluster)  [unwired: 8 in, 1 out]
  n192 = Merge Errors(w140, w139, w138, w137, w64, w318, w317, w63, w62, w61, w313, w312, w311, w310) -> (w316:errorcluster)
  n193 = call-dynamic "close context.vi"("error in (no error)"=w316, "Socket in"=w315) -> ("error out"=→"error out":errorcluster)  [unwired: 8 in, 1 out]
